vi "OAT Reconstruct Order Waveform.vi"(5 "reset? (TRUE)":bool=TRUE, 6 "unit in degree? (F)":bool, 7 "order":dbl=1.0 format="%.2f", 8 "samples/revolution wanted":dbl=4.0 format="%.2f", 9 "samples/revolution":dbl=1.0 format="%.2f", 10 "phase lag":dbl[](array[numeric]) format="%.2f", 11 "magnitude":dbl[](array[numeric]) format="%.2f") -> (0 "error out":errorcluster, 2 "actual samples/rev":dbl=1.0 format="%.2f", 3 "order waveform":dbl[](array[numeric]) format="%.2f")   [LabVIEW 2017, in "SoundVib_Resampling.lvlib"]
uses:
  <vilib>/addons/Sound and Vibration/Order Analysis/Resample Order Tracking/SoundVib_Resampling.lvlib
  <vilib>/Analysis/NI_AALPro.lvlib
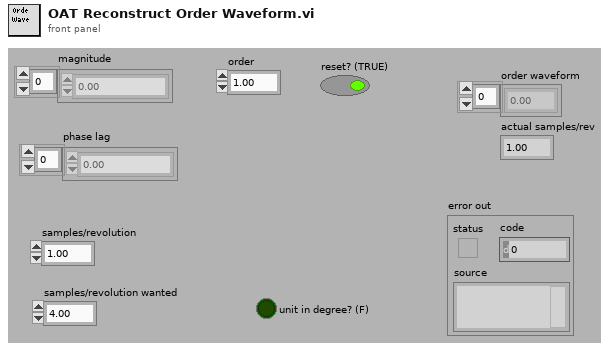
[diagram p1: front panel]
types:
  T1 = typedef "OAT Decimation Filter.ctl" = cluster{"coefficients":dbl[], "factor":i32}
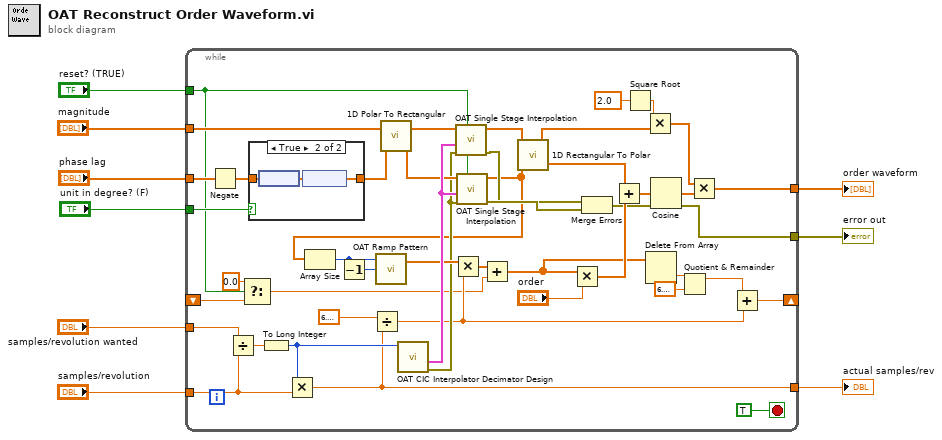
[diagram p0: block diagram]
diagram:
  n1 = while {
    tunnel: "samples/revolution wanted" -> [w54]
    tunnel: "samples/revolution" -> [w51]
    tunnel: [w38] -> w7
    tunnel: "magnitude" -> [w35]
    tunnel: "unit in degree? (F)" -> [w14]
    tunnel: [w28] -> w4
    tunnel: [w26] -> w3
    tunnel: "phase lag" -> [w25]
    shift-right: [w18] -> _
    shift-left: _ -> [w15]
    tunnel: "reset? (TRUE)" -> [w10]
    stop <- TRUE stop-if-true
    n2 = Negate(x=w25) -> (-x=w32:dbl[])
    n3 = Divide(x=w54, y=w51) -> (x/y=w53:dbl)
    n4 = Select(t=0.0, s=w10, f=w15) -> (s? t:f=w12:dbl)
    n5 = case shown="True" w14 {
      tunnel: w32 -> [w55 w58]
      tunnel: [w55 w56] -> w33
      frame False {
      }
      frame True {
        n6 = node(w58) -> (w57:dbl[unit][])
        n7 = node(w57) -> (w56:dbl[])
      }
    }
    n8 = To Long Integer(number=w53) -> (32bit integer=w46:i32)
    n9 = Multiply(x=w46, y=w51) -> (x*y=w26:dbl)
    n10 = Divide(x=6.283185307179586, y=w26) -> (x/y=w19:dbl)
    n11 = call <vilib>:"1D Polar To Rectangular.vi"("Magnitude"=w35, "Phase"=w33) -> ("X"=w37:dbl[], "Y"=w36:dbl[])  [unwired: 1 out]
    n12 = call <vilib>:"OAT CIC Interpolator Decimator Design.vi"("interpolation/decimation factor"=w46) -> ("error out"=w31:errorcluster, "filter"=w52:T1)  [unwired: 9 in]
    n13 = call <vilib>:"OAT Single Stage Interpolation.vi"("reset? (True)"=w10, "error in (no error)"=w31, "filter"=w52, "X"=w37) -> ("error out"=w29:errorcluster, "Y"=w42:dbl[])  [unwired: 6 in]
    n14 = call <vilib>:"OAT Single Stage Interpolation.vi"("reset? (True)"=w10, "error in (no error)"=w31, "filter"=w52, "X"=w36) -> ("error out"=w30:errorcluster, "Y"=w24:dbl[])  [unwired: 6 in]
    n15 = Array Size(array=w24) -> (size(s)=w11:i32)
    n16 = Decrement(x=w11) -> (x-1=w50:i32)
    n17 = call <vilib>:"OAT Ramp Pattern.vi"("end"=w50, "samples"=w11) -> ("Ramp Pattern"=w39:dbl[])  [unwired: 1 in, 1 out]
    n18 = Multiply(x=w39, y=w19) -> (x*y=w17:dbl[])
    n19 = Add(x=w17, y=w12) -> (x+y=w16:dbl[])
    n20 = call <vilib>:"1D Rectangular To Polar.vi"("X"=w42, "Y"=w24) -> ("Magnitude"=w40:dbl[], "Phase"=w41:dbl[])  [unwired: 1 out]
    n21 = Multiply(x=w16, y="order") -> (x*y=w45:dbl[])
    n22 = Merge Errors(w29, w30) -> (w28:errorcluster)
    n23 = Add(x=w41, y=w45) -> (x+y=w44:dbl[])
    n24 = Square Root(x=2.0) -> (sqrt(x)=w48:dbl)
    n25 = Multiply(x=w48, y=w40) -> (x*y=w27:dbl[])
    n26 = Delete From Array(array=w16) -> (deleted portion=w22:dbl)  [unwired: 2 in, 1 out]
    n27 = Cosine(x=w44) -> (cos(x)=w43:dbl[])
    n28 = Quotient & Remainder(x=w22, y=6.283185307179586) -> (x-y*floor(x/y)=w20:dbl)  [unwired: 1 out]
    n29 = Multiply(x=w27, y=w43) -> (x*y=w38:dbl[])
    n30 = Add(x=w20, y=w19) -> (x+y=w18:dbl)
  }
  "order waveform" <- w7
  "actual samples/rev" <- w3
  "error out" <- w4
